vi "MyGlobals.vi"() -> ()   [LabVIEW 2012]
panel:
  out "gSlave3Text":string
  out "gSlave2Text":string
  out "gSlave1Text":string
  out "gMasterText":string
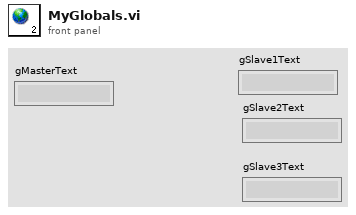
[diagram p1: front panel]
diagram:
